vi "SubVI_FullRampDrive_Teleop.vi"(11 "Y Axis Input":dbl) -> (3 "Y Axis Output":dbl)   [LabVIEW 2017]
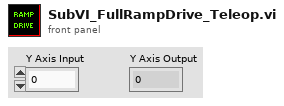
[diagram p1: front panel]
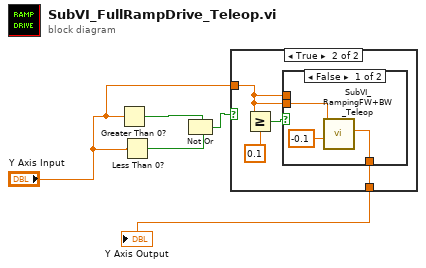
[diagram p0: block diagram]
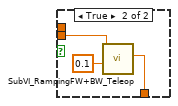
[diagram p3: hidden frame]
diagram:
  n1 = Greater Than 0?(x="Y Axis Input") -> (x > 0?=w2:bool)
  n2 = Less Than 0?(x="Y Axis Input") -> (x < 0?=w1:bool)
  n3 = Not Or(1:w1, 2:w2) -> (0:w4:bool)
  n4 = case shown="True" w4 {
    tunnel: "Y Axis Input" -> [w6 w8]
    tunnel: [w6 w7] -> w5
    frame False {
    }
    frame True {
      n5 = Greater Or Equal?(x=w8, y=0.1) -> (x >= y?=w9:bool)
      n6 = case shown="False" w9 {
        tunnel: w8 -> [_ _]
        tunnel: w8 -> [w13 w16]
        tunnel: [w11 w14] -> w7
        frame False {
          n7 = call "SubVI_RampingFW+BW_Teleop.vi"("+Speed/s"=-0.1, "Y Axis Input(Changing Value)"=w13) -> ("Y Axis Output"=w11:dbl)  [unwired: 9 in]
        }
        frame True {
          n8 = call "SubVI_RampingFW+BW_Teleop.vi"("+Speed/s"=0.1, "Y Axis Input(Changing Value)"=w16) -> ("Y Axis Output"=w14:dbl)  [unwired: 9 in]
        }
      }
    }
  }
  "Y Axis Output" <- w5
